vi "Aquisicao.vi"() -> ()   [LabVIEW 2014]
panel:
  in  "Slide":dbl(slide) scale=0.0..5.0
  out "Vibracao":dbl
  out "Celula":dbl
  out "Rotacao":dbl
  out "TermoparRef":dbl
  out "Termopar 2":dbl
  out "Termopar 1":dbl
  in  "stop":bool
  out "Vibracao":dynamicdata(graph)
  in  "Freio":bool
  in  "Motor":bool
  out "Freio":bool
  out "Motor":bool
  out "Célula":dynamicdata(graph)
  out "Rotação":dynamicdata(graph)
  out "Termopar 2":dynamicdata(graph)
  out "Termopar Ref":dynamicdata(graph)
  out "Termopar 1":dynamicdata(graph)
  # "Bancada de Frenagem -  Calibração"
  # "Valores Gráficos"
  # "Numérico"
  # "Acionamento"
  # "Controle"
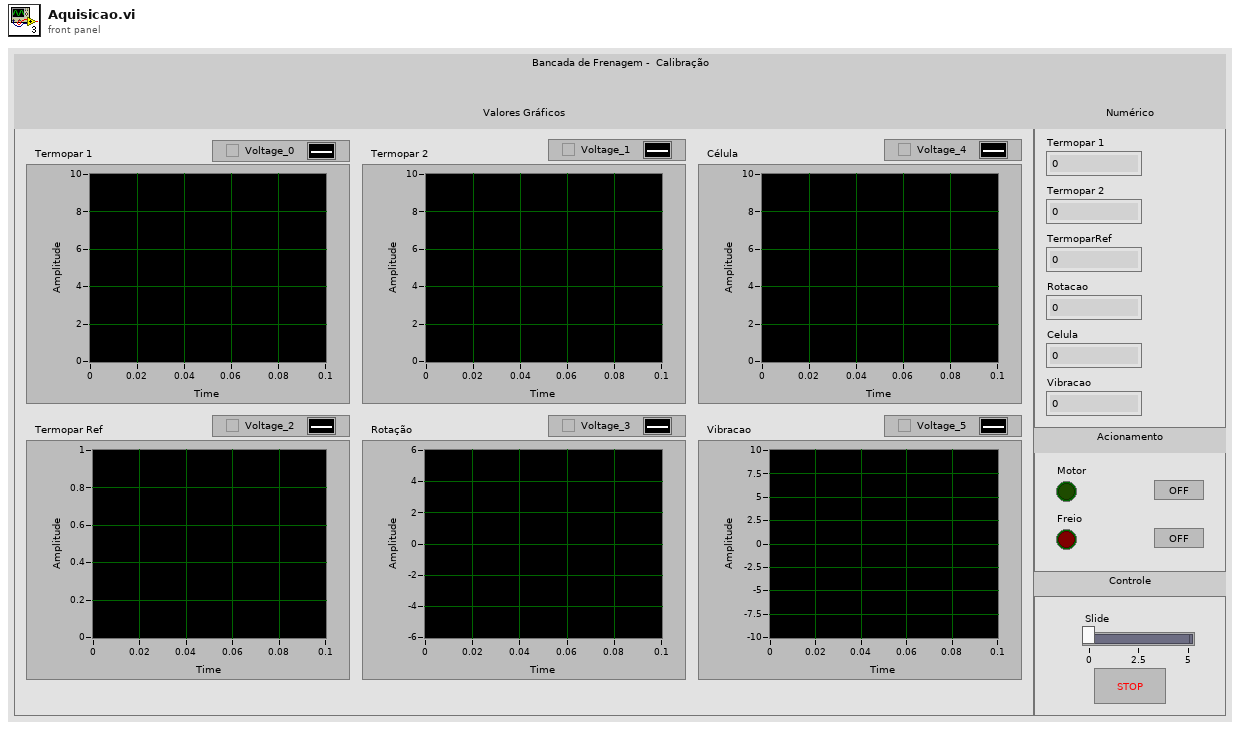
[diagram p1: front panel]
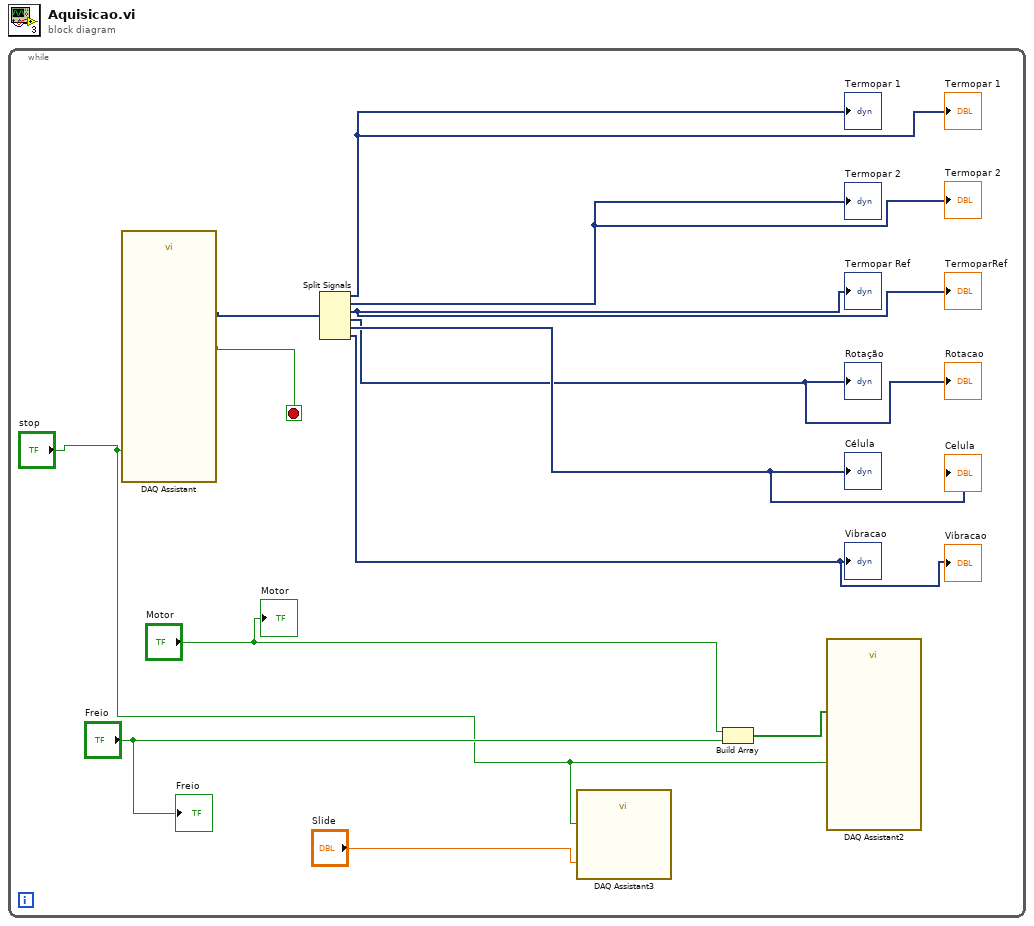
[diagram p0: block diagram]
diagram:
  n1 = while {
    stop <- w2 stop-if-true
    n2 = call "DAQ Assistant"("stop (F)"="stop") -> ("data"=w3:dynamicdata, "stopped"=w2:bool)  [unwired: 15 in, 2 out]
    n3 = Split Signals(w3) -> (→"Termopar 1" →"Termopar 1":dynamicdata, →"Termopar 2" →"Termopar 2":dynamicdata, →"Termopar Ref" →"TermoparRef":dynamicdata, →"Rotação" →"Rotacao":dynamicdata, →"Célula" →"Celula":dynamicdata, →"Vibracao" →"Vibracao":dynamicdata)  [unwired: 6 in]
    n4 = call "DAQ Assistant3"("data"="Slide", "stop (T)"="stop") -> ()  [unwired: 16 in, 2 out]
    n5 = Build Array("Motor", "Freio") -> (w7:bool[])
    n6 = call "DAQ Assistant2"("data"=w7, "stop (T)"="stop") -> ()  [unwired: 16 in, 2 out]
    "Motor" <- "Motor"
    "Freio" <- "Freio"
  }
